vi "Tree_FocusArrayTag_Tests.vi"(11 "error in":errorcluster) -> (15 "error out":errorcluster)   [LabVIEW 2016, in "DronaTest.lvlib"]
uses:
  DronaTest.lvlib
  APIs/Stimulus/ControlValue/SetValueAuto.vi
  APIs/Stimulus/ControlValue/Controls/Tree/SetValueByItemTagArray.vi
  APIs/Assert/AssertControlValue/Controls/Tree/AssertValueByArrayTags.vi
  <vilib>/addons/_JKI Toolkits/Caraya/classes/Assert/Assert Equal Value_Variant.vi
  <vilib>/addons/_JKI Toolkits/Caraya/classes/Assert/Assert Error.vi
  <vilib>/addons/_JKI Toolkits/Caraya/classes/Test/Test.lvclass
  Drona.lvlib
  <vilib>/SLL Toolkit/SLL Debug/SLL Debug.lvlib
  APIs/Stimulus/ControlValue/ControlValue.lvlib
  <vilib>/addons/_JKI Toolkits/Caraya/classes/Assert/Assert.lvclass
  APIs/Stimulus/ControlValue/Controls/Tree/StimulusTree.lvlib
  APIs/Assert/AssertControlValue/Controls/Tree/AssertTree.lvlib
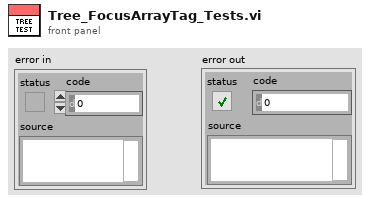
[diagram p1: front panel]
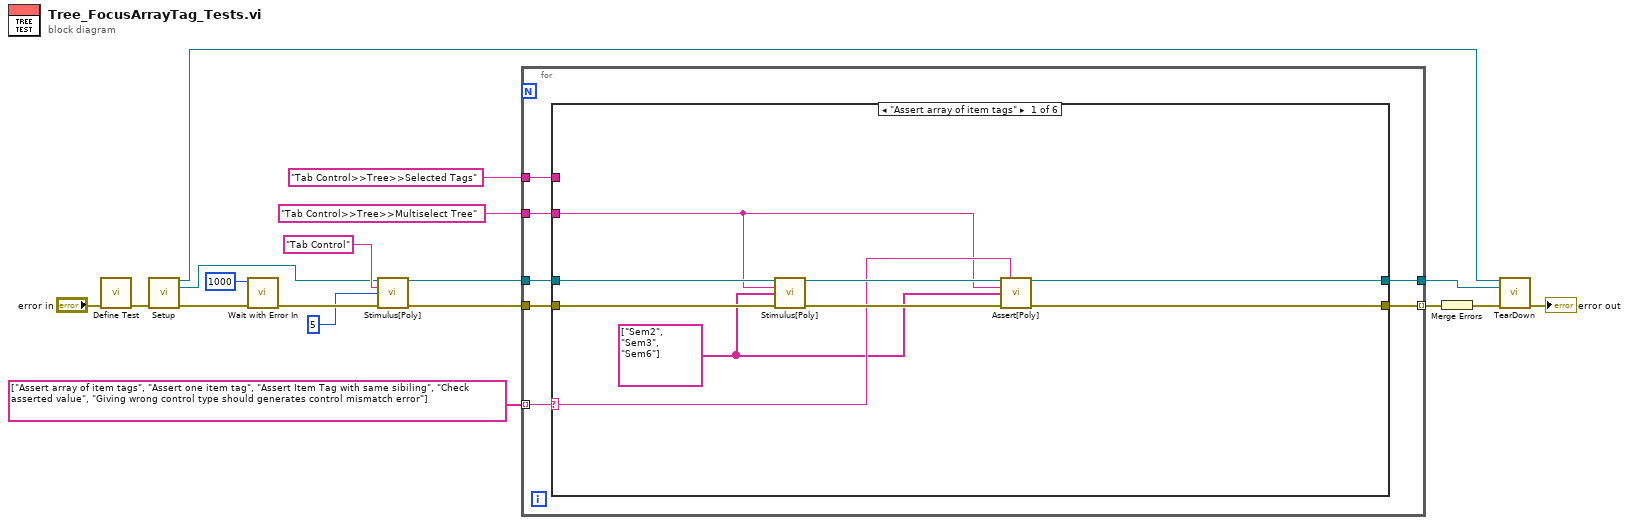
[diagram p0: block diagram]
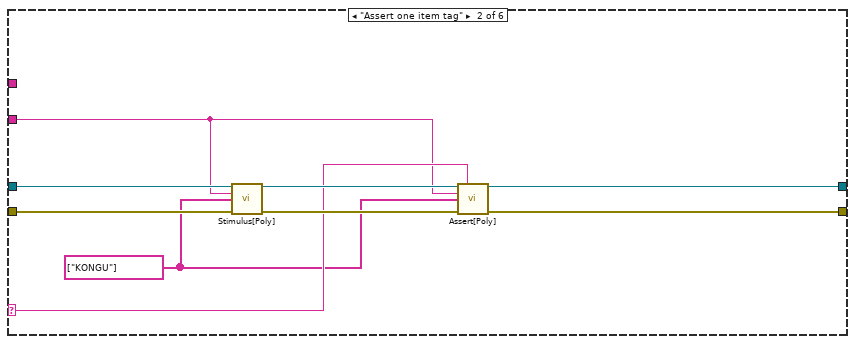
[diagram p2: hidden frame]
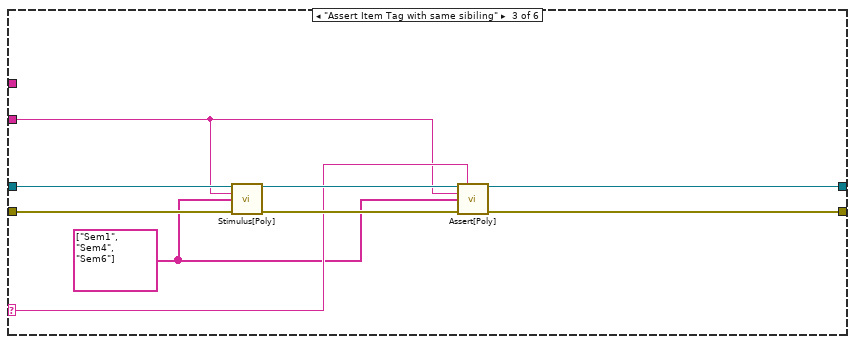
[diagram p3: hidden frame]
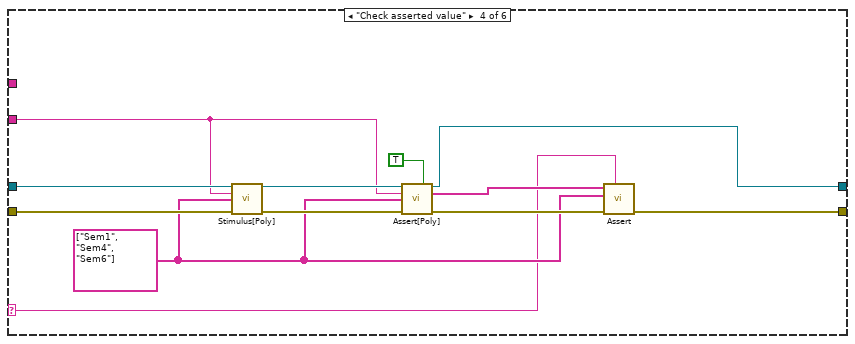
[diagram p4: hidden frame]
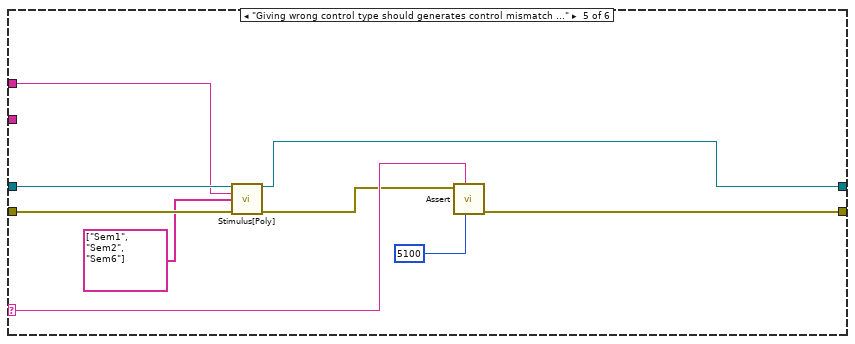
[diagram p5: hidden frame]
diagram:
  n1 = call <vilib>:"Define Test.vi"("error in (no error)"="error in") -> ("error out"=w7:errorcluster)  [unwired: 9 in, 1 out]
  n2 = call "Setup.vi"("error in (no error)"=w7) -> ("Application Ref"=w2:refnum<vi>, "VI out"=w6:refnum<vi>, "error out"=w5:errorcluster)  [unwired: 12 in]
  n3 = call <vilib>:"Wait with Error In.vi"("error in (no error)"=w5, "milliseconds to wait"=u32 1000) -> ("error out"=w16:errorcluster)  [unwired: 9 in]
  n4 = call-poly "Stimulus[Poly].vi"("VI Reference In"=w6, "Control Path"="Tab Control", "Value (Signaling)"=5, "error in"=w16) -> ("VI Reference Out"=w12:refnum<vi>, "error out"=w15:errorcluster)  [unwired: 10 in]
  n5 = for {
    tunnel: w12 -> [w24]
    tunnel: "Tab Control>>Tree>>Multiselect Tree" ("Control Path") -> [w23]
    tunnel: "Tab Control>>Tree>>Selected Tags" ("Control Path") -> [w22]
    tunnel: string[] ["Assert array of item tags", "Assert one item tag", "Assert Item Tag with same sibiling", "Check asserted value", "Giving wrong control type should generates control mismatch error"] -> [w20] mode=indexing
    tunnel: [w19] -> w3
    tunnel: w15 -> [w25]
    tunnel: [w21] -> w8 mode=indexing
    n6 = case shown="\"Assert array of item tags\"" w20 {
      selector: w20 -> [w28 w37 w46 w55 w70 _]
      tunnel: w25 -> [w34 w43 w52 w64 w73 w75]
      tunnel: w24 -> [w33 w42 w51 w63 w72 w74]
      tunnel: w23 -> [w26 w35 w44 w60 _ _]
      tunnel: w22 -> [_ _ _ _ w66 _]
      tunnel: [w30 w39 w48 w54 w71 w75] -> w21
      tunnel: [w29 w38 w47 w53 w69 w74] -> w19
      frame "Assert array of item tags" {
        w27 = string[] ["Sem2", "Sem3", "Sem6"] ("Item Name")
        n7 = call-poly "Stimulus[Poly].vi"("VI Reference In"=w33, "Control Path"=w26, "Item Tags Array"=w27, "Error In"=w34) -> ("VI Reference Out"=w31:refnum<vi>, "Error Out"=w32:errorcluster)  [unwired: 10 in]
        n8 = call-poly "Assert[Poly].vi"("VI Reference In"=w31, "Test Label"=w28, "Control Path"=w26, "Focus Item Tag"=w27, "Error In"=w32) -> ("VI Reference Out"=w29:refnum<vi>, "Error Out"=w30:errorcluster)  [unwired: 8 in, 1 out]
      }
      frame "Assert one item tag" {
        w36 = string[] ["KONGU"] ("Item Name")
        n9 = call-poly "Stimulus[Poly].vi"("VI Reference In"=w42, "Control Path"=w35, "Item Tags Array"=w36, "Error In"=w43) -> ("VI Reference Out"=w40:refnum<vi>, "Error Out"=w41:errorcluster)  [unwired: 10 in]
        n10 = call-poly "Assert[Poly].vi"("VI Reference In"=w40, "Test Label"=w37, "Control Path"=w35, "Focus Item Tag"=w36, "Error In"=w41) -> ("VI Reference Out"=w38:refnum<vi>, "Error Out"=w39:errorcluster)  [unwired: 8 in, 1 out]
      }
      frame "Assert Item Tag with same sibiling" {
        w45 = string[] ["Sem1", "Sem4", "Sem6"] ("Item Name")
        n11 = call-poly "Stimulus[Poly].vi"("VI Reference In"=w51, "Control Path"=w44, "Item Tags Array"=w45, "Error In"=w52) -> ("VI Reference Out"=w49:refnum<vi>, "Error Out"=w50:errorcluster)  [unwired: 10 in]
        n12 = call-poly "Assert[Poly].vi"("VI Reference In"=w49, "Test Label"=w46, "Control Path"=w44, "Focus Item Tag"=w45, "Error In"=w50) -> ("VI Reference Out"=w47:refnum<vi>, "Error Out"=w48:errorcluster)  [unwired: 8 in, 1 out]
      }
      frame "Check asserted value" {
        w56 = string[] ["Sem1", "Sem4", "Sem6"] ("Item Name")
        n13 = call-poly "Stimulus[Poly].vi"("VI Reference In"=w63, "Control Path"=w60, "Item Tags Array"=w56, "Error In"=w64) -> ("VI Reference Out"=w61:refnum<vi>, "Error Out"=w62:errorcluster)  [unwired: 10 in]
        n14 = call-poly "Assert[Poly].vi"("VI Reference In"=w61, "Assert Only? (F)"=TRUE, "Control Path"=w60, "Focus Item Tag"=w56, "Error In"=w62) -> ("VI Reference Out"=w53:refnum<vi>, "Asserted Value"=w57:string[], "Error Out"=w58:errorcluster)  [unwired: 8 in]
        n15 = call-poly <vilib>:"Assert.vi"("Label"=w55, "error in (no error)"=w58, "Y"=w56, "X"=w57) -> ("error out"=w54:errorcluster)  [unwired: 6 in, 1 out]
      }
      frame "Giving wrong control type should generates control mismatch error" {
        n16 = call-poly "Stimulus[Poly].vi"("VI Reference In"=w72, "Control Path"=w66, "Item Tags Array"=string[] ["Sem1", "Sem2", "Sem6"] ("Item Name"), "Error In"=w73) -> ("VI Reference Out"=w69:refnum<vi>, "Error Out"=w68:errorcluster)  [unwired: 10 in]
        n17 = call-poly <vilib>:"Assert.vi"("error code (1)"=5100, "Label"=w70, "Error?"=w68) -> ("error out"=w71:errorcluster)  [unwired: 7 in, 1 out]
      }
      frame Default {
      }
    }
  }
  n18 = Merge Errors(w8) -> (w4:errorcluster)
  n19 = call "TearDown.vi"("Application Ref"=w2, "VI in"=w3, "error in (no error)"=w4) -> ("error out"=→"error out":errorcluster)  [unwired: 12 in]
